vi "Scenes.vi"(8 "error in (no error)":errorcluster, 11 "RGetSceneList in":refnum<class "RGetSceneList.lvclass">) -> (0 "error out":errorcluster, 1 "Preview Scene":string, 2 "Program Scene":string, 3 "RGetSceneList out":refnum<class "RGetSceneList.lvclass">, 4 "Scenes":T1[](array[typedef]))   [LabVIEW 2022 SP3, in "obs-websocket-lv.lvlib" / "RGetSceneList.lvclass"]
uses:
  RGetSceneList.lvclass
  RGetSceneList.lvclass/RGetSceneList.ctl
  Scene.ctl
  obs-websocket-lv.lvlib
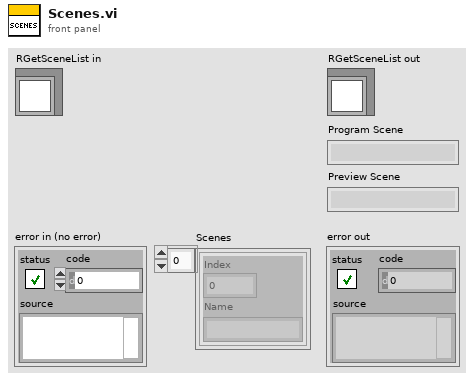
[diagram p1: front panel]
types:
  T1 = typedef "obs-websocket-lv.lvlib/Scene.ctl" = cluster{"Index":i32, "Name":string}
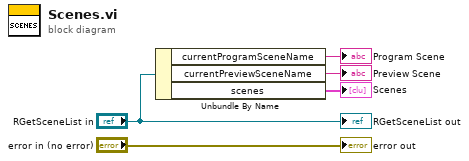
[diagram p0: block diagram]
diagram:
  n1 = Unbundle By Name("RGetSceneList in") -> ("currentProgramSceneName"=→"Program Scene":string, "currentPreviewSceneName"=→"Preview Scene":string, "scenes"=→"Scenes":T1[])
  "error out" <- "error in (no error)"
  "RGetSceneList out" <- "RGetSceneList in"
